vi "FlatToRichnixnet_grpc_ReadFrameRequest.vi"(5 "OutputClusterType":T1, 11 "InputCluster":T3) -> (3 "OutputCluster":T1)   [LabVIEW 2025, in "xnet-grpc_client.lvlib"]
uses:
  nixnet_grpc_ReadFrameRequest_Flat.ctl
  nidevice_grpc_Session_Flat.ctl
  nixnet_grpc_Protocol.ctl
  nixnet_grpc_TimeOut.ctl
  nixnet_grpc_ReadFrameRequest.ctl
  nixnet_grpc_ReadFrameRequest_protocol_enum/nixnet_grpc_ReadFrameRequest_protocol_enum.lvclass
  nixnet_grpc_ReadFrameRequest_timeout_enum/nixnet_grpc_ReadFrameRequest_timeout_enum.lvclass
  nidevice_grpc_Session.ctl
  xnet-grpc_client.lvlib
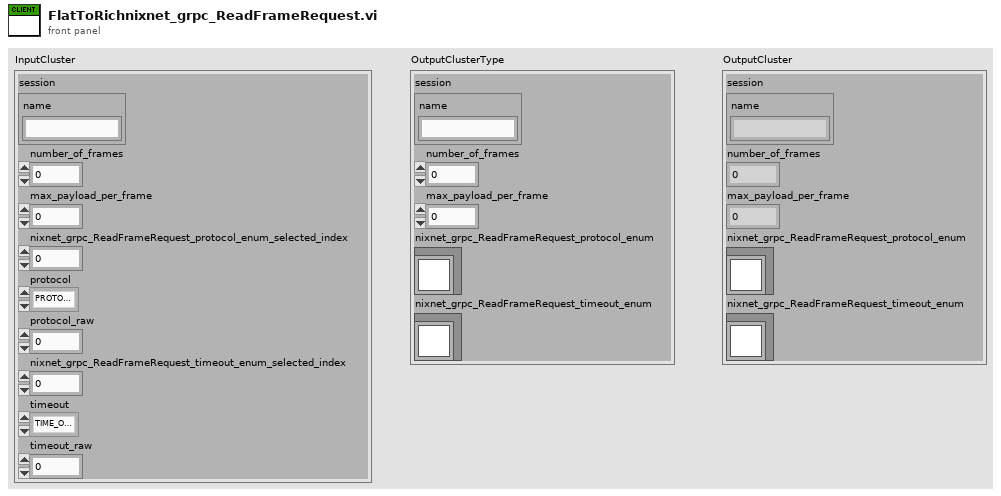
[diagram p1: front panel]
types:
  T1 = typedef "xnet-grpc_client.lvlib/nixnet_grpc_ReadFrameRequest.ctl" = cluster{"session":T2, "number_of_frames":i32, "max_payload_per_frame":u32, "nixnet_grpc_ReadFrameRequest_protocol_enum":refnum<class "nixnet_grpc_ReadFrameRequest_protocol_enum.lvclass">, "nixnet_grpc_ReadFrameRequest_timeout_enum":refnum<class "nixnet_grpc_ReadFrameRequest_timeout_enum.lvclass">}
  T2 = typedef "xnet-grpc_client.lvlib/nidevice_grpc_Session.ctl" = cluster{"name":string}
  T3 = typedef "xnet-grpc_client.lvlib/nixnet_grpc_ReadFrameRequest_Flat.ctl" = cluster{"session":T4, "number_of_frames":i32, "max_payload_per_frame":u32, "nixnet_grpc_ReadFrameRequest_protocol_enum_selected_index":i32, "protocol":T5, "protocol_raw":u32, "nixnet_grpc_ReadFrameRequest_timeout_enum_selected_index":i32, "timeout":T6, "timeout_raw":dbl}
  T4 = typedef "xnet-grpc_client.lvlib/nidevice_grpc_Session_Flat.ctl" = cluster{"name":string}
  T5 = typedef "xnet-grpc_client.lvlib/nixnet_grpc_Protocol.ctl" = enum32{"PROTOCOL_UNSPECIFIED", "PROTOCOL_CAN", "PROTOCOL_LIN", "PROTOCOL_FLEX_RAY", "PROTOCOL_J1939", "PROTOCOL_ENET"}
  T6 = typedef "xnet-grpc_client.lvlib/nixnet_grpc_TimeOut.ctl" = enum32{"TIME_OUT_NONE", "TIME_OUT_INFINITE"}
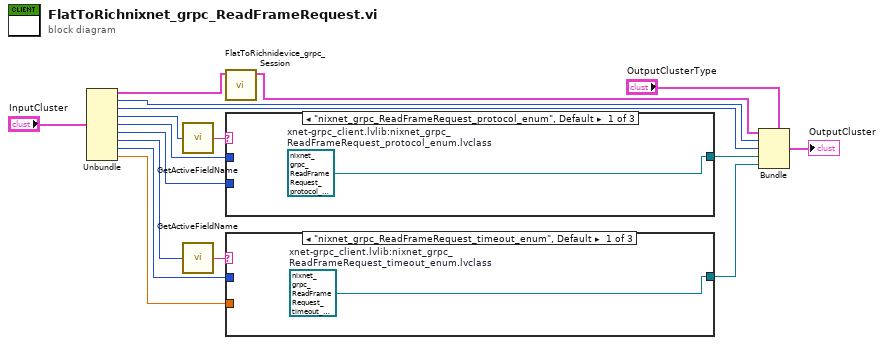
[diagram p0: block diagram]
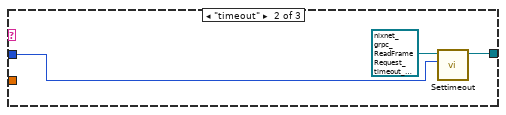
[diagram p2: hidden frame]
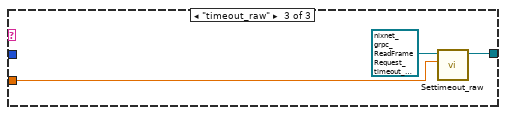
[diagram p3: hidden frame]
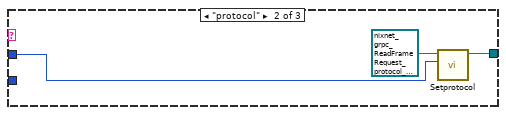
[diagram p4: hidden frame]
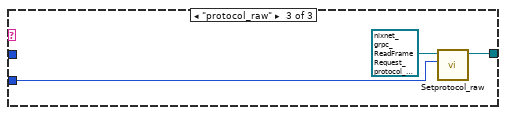
[diagram p5: hidden frame]
diagram:
  n1 = Unbundle "Unbundle"("InputCluster") -> ("session"=w14:T4, "number_of_frames"=w12:i32, "max_payload_per_frame"=w11:u32, "nixnet_grpc_ReadFrameRequest_protocol_enum_selected_index"=w10:i32, "protocol"=w7:T5, "protocol_raw"=w6:u32, "nixnet_grpc_ReadFrameRequest_timeout_enum_selected_index"=w5:i32, "timeout"=w2:T6, "timeout_raw"=w1:dbl)
  n2 = call "GetActiveFieldName.vi"("protobuf index"=w10) -> ("oneof field name"=w9:string)
  n3 = call "GetActiveFieldName.vi"("protobuf index"=w5) -> ("oneof field name"=w4:string)
  n4 = call "FlatToRichnidevice_grpc_Session.vi"("InputCluster"=w14) -> ("OutputCluster"=w13:T2)  [unwired: 10 in]
  n5 = case "nixnet_grpc_ReadFrameRequest_protocol_enum" shown="\"nixnet_grpc_ReadFrameRequest_protocol_enum\", Default" w9 {
    tunnel: [w18 w20 w23] -> w8
    tunnel: w7 -> [_ w21 _]
    tunnel: w6 -> [_ _ w24]
    frame "nixnet_grpc_ReadFrameRequest_protocol_enum", Default {
      w18 = refnum<class "nixnet_grpc_ReadFrameRequest_protocol_enum.lvclass"> refnum  # xnet-grpc_client.lvlib:nixnet_grpc_ReadFrameRequest_protocol_enum.lvclass
    }
    frame "protocol" {
      n6 = call "Setprotocol.vi"("Set_Val"=w21, "OneOfTemplate in"=refnum<class "nixnet_grpc_ReadFrameRequest_protocol_enum.lvclass"> refnum) -> ("OneOfTemplate out"=w20:refnum<class "nixnet_grpc_ReadFrameRequest_protocol_enum.lvclass">)  [unwired: 8 in, 1 out]
    }
    frame "protocol_raw" {
      n7 = call "Setprotocol_raw.vi"("Set_Val"=w24, "OneOfTemplate in"=refnum<class "nixnet_grpc_ReadFrameRequest_protocol_enum.lvclass"> refnum) -> ("OneOfTemplate out"=w23:refnum<class "nixnet_grpc_ReadFrameRequest_protocol_enum.lvclass">)  [unwired: 8 in, 1 out]
    }
  }
  n8 = case "nixnet_grpc_ReadFrameRequest_timeout_enum" shown="\"nixnet_grpc_ReadFrameRequest_timeout_enum\", Default" w4 {
    tunnel: [w25 w27 w30] -> w3
    tunnel: w2 -> [_ w28 _]
    tunnel: w1 -> [_ _ w31]
    frame "nixnet_grpc_ReadFrameRequest_timeout_enum", Default {
      w25 = refnum<class "nixnet_grpc_ReadFrameRequest_timeout_enum.lvclass"> refnum  # xnet-grpc_client.lvlib:nixnet_grpc_ReadFrameRequest_timeout_enum.lvclass
    }
    frame "timeout" {
      n9 = call "Settimeout.vi"("Set_Val"=w28, "OneOfTemplate in"=refnum<class "nixnet_grpc_ReadFrameRequest_timeout_enum.lvclass"> refnum) -> ("OneOfTemplate out"=w27:refnum<class "nixnet_grpc_ReadFrameRequest_timeout_enum.lvclass">)  [unwired: 8 in, 1 out]
    }
    frame "timeout_raw" {
      n10 = call "Settimeout_raw.vi"("Set_Val"=w31, "OneOfTemplate in"=refnum<class "nixnet_grpc_ReadFrameRequest_timeout_enum.lvclass"> refnum) -> ("OneOfTemplate out"=w30:refnum<class "nixnet_grpc_ReadFrameRequest_timeout_enum.lvclass">)  [unwired: 8 in, 1 out]
    }
  }
  n11 = Bundle "Bundle"(cluster="OutputClusterType", "session"=w13, "number_of_frames"=w12, "max_payload_per_frame"=w11, "nixnet_grpc_ReadFrameRequest_protocol_enum"=w8, "nixnet_grpc_ReadFrameRequest_timeout_enum"=w3) -> (→"OutputCluster":T1)
